vi "CAENHV Get Bd Param Prop.vi"(7 "PropName":string, 8 "error in (no error)":errorcluster, 9 "ParName":string, 10 "slot":u16, 11 "handle":i32) -> (0 "error out":errorcluster, 3 "retval":u32)   [LabVIEW 2018, in "CAENHVWrapper.lvlib"]
doc: "CAENHVLIB_API CAENHVRESULT CAENHV_GetBdParamProp(int handle, \n ushort slot, const char *ParName, const char *PropName, void *retval);"
uses:
  <instrlib>/CAENHVWrapper/CAENHVWrapper.lvlib
  <instrlib>/CAENHVWrapper/VIs/CAENHVWrapper.dll
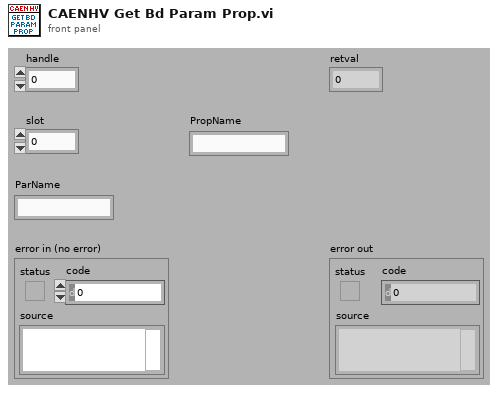
[diagram p1: front panel]
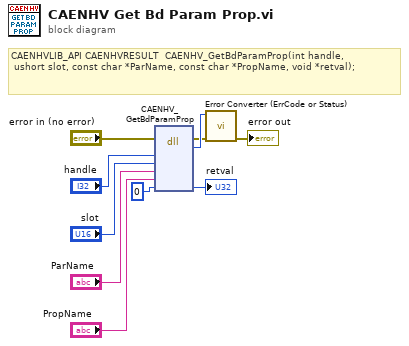
[diagram p0: block diagram]
diagram:
  # "CAENHVLIB_API CAENHVRESULT  CAENHV_GetBdParamProp(int handle, \n ushort slot, const char *ParName, const char *PropName, void *retval);"
  n1 = dll-call lib="C:/Program Files (x86)/National Instruments/LabVIEW 2018/instr.lib/CAENHVWrapper/VIs/CAENHVWrapper.*" fn="CAENHV_GetBdParamProp"(error in="error in (no error)", "handle"="handle", "slot"="slot", "ParName"="ParName", "PropName"="PropName", "retval"=u32 0) -> (error out=w2:errorcluster, "return type"=w3:i32, "retval"=→"retval":u32)  [unwired: 6 in, 1 out]
  n2 = call <instrlib>:"Error Converter (ErrCode or Status).vi"("error in (no error)"=w2, "error code"=w3) -> ("error out"=→"error out":errorcluster)  [unwired: 9 in]
